vi "Visualisation.vi"() -> ()   [LabVIEW 2020]
panel:
  out "Boolean 2":bool
  out "Boolean":bool
  out "Gauge 2":dbl(knob) scale=0.0..180.0
  out "error out":errorcluster {"code" format="%.0b"}
  out "Light Left":string
  out "Gauge":dbl(knob) scale=0.0..180.0
  out "Light Right":string
  out "Angle Right":string
  in  "stop":bool
  out "Angle Left":string
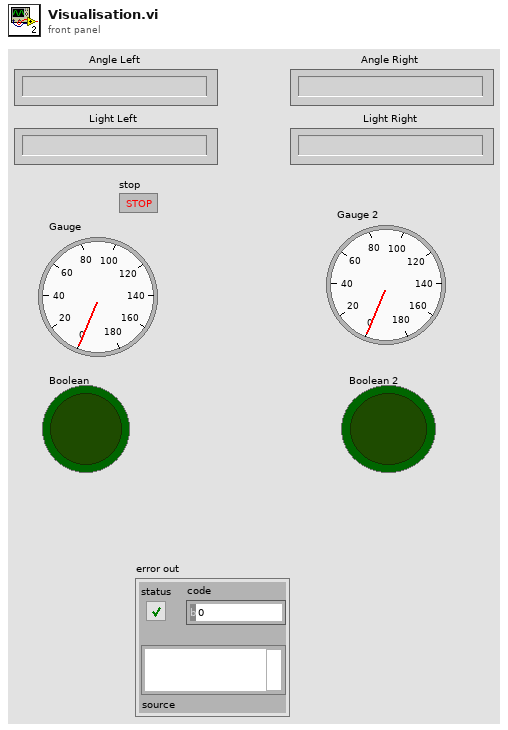
[diagram p1: front panel]
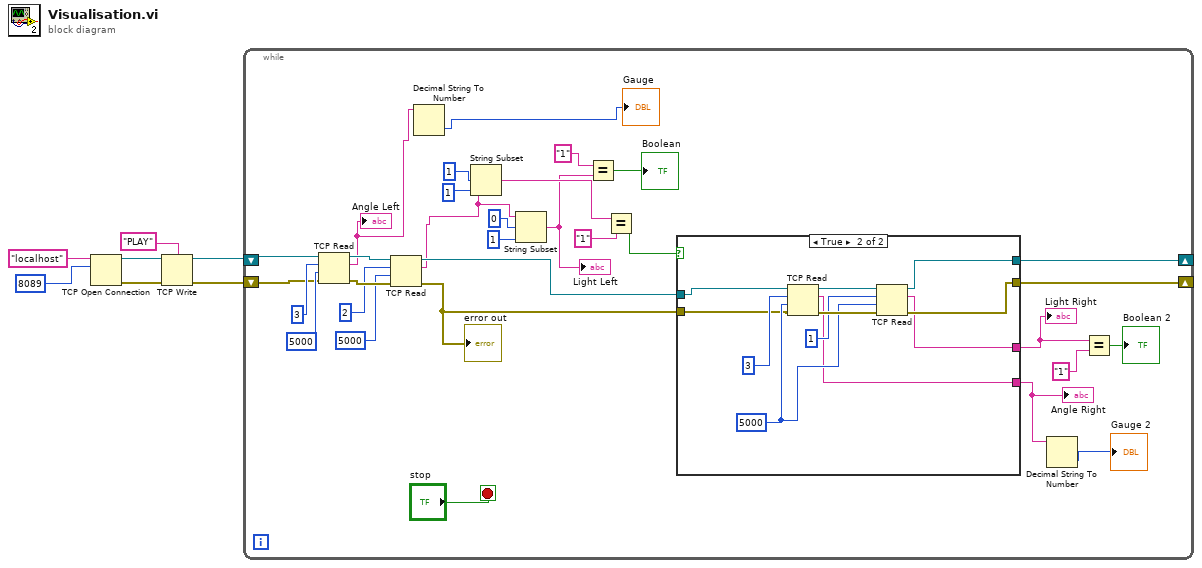
[diagram p0: block diagram]
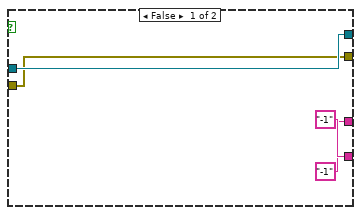
[diagram p2: hidden frame]
diagram:
  n1 = TCP Open Connection(address="localhost", remote port or service name=u16 8089) -> (connection ID=w5:refnum<k5>, error out=w4:errorcluster)  [unwired: 3 in]
  n2 = TCP Write(connection ID=w5, data in="PLAY", error in (no error)=w4) -> (connection ID out=w3:refnum<k5>, error out=w2:errorcluster)  [unwired: 1 in, 1 out]
  n3 = while {
    shift-right: [w23] -> _
    shift-left: w3 -> [w36]
    shift-right: [w22] -> _
    shift-left: w2 -> [w35]
    stop <- "stop" stop-if-true
    n4 = TCP Read(connection ID=w36, bytes to read=3, error in (no error)=w35, 9:5000 ("timeout ms (25000)")) -> (connection ID out=w33:refnum<k5>, data out=w21:string, error out=w32:errorcluster)  [unwired: 1 in]
    "Angle Left" <- w21
    n5 = TCP Read(connection ID=w33, bytes to read=2, error in (no error)=w32, 9:5000 ("timeout ms (25000)")) -> (connection ID out=w24:refnum<k5>, data out=w17:string, error out=w15:errorcluster)  [unwired: 1 in]
    "error out" <- w15
    n6 = Decimal String To Number(string=w21) -> (number=→"Gauge":i32)  [unwired: 2 in, 1 out]
    n7 = String Subset(string=w17, offset (0)=1, length (rest)=1 ("length (rest)")) -> (substring=w27:string)
    n8 = String Subset(string=w17, offset (0)=0, length (rest)=1 ("length (rest)")) -> (substring=w13:string)
    "Light Left" <- w13
    n9 = Equal?(x="1" ("y"), y=w13) -> (x = y?=→"Boolean":bool)
    n10 = Equal?(x=w27, y="1") -> (x = y?=w26:bool)
    n11 = case shown="True" w26 {
      tunnel: w24 -> [w42 w48]
      tunnel: w15 -> [w41 w47]
      tunnel: [w42 w46] -> w23
      tunnel: [w41 w45] -> w22
      tunnel: ["-1" ("data out") w43] -> w10
      tunnel: ["-1" ("data out") w44] -> w16
      frame False {
      }
      frame True {
        w49 = 5000 ("timeout ms (25000)")
        n12 = TCP Read(connection ID=w48, bytes to read=3, error in (no error)=w47, 9:w49) -> (connection ID out=w52:refnum<k5>, data out=w44:string, error out=w53:errorcluster)  [unwired: 1 in]
        n13 = TCP Read(connection ID=w52, bytes to read=1, error in (no error)=w53, 9:w49) -> (connection ID out=w46:refnum<k5>, data out=w43:string, error out=w45:errorcluster)  [unwired: 1 in]
      }
    }
    "Angle Right" <- w16
    "Light Right" <- w10
    n14 = Decimal String To Number(string=w16) -> (number=→"Gauge 2":i32)  [unwired: 2 in, 1 out]
    n15 = Equal?(x=w10, y="1") -> (x = y?=→"Boolean 2":bool)
  }
